vi "Get Key-Value Pairs from Attribute List.vi"(7 "element name (for errors)":string, 8 "error in (no error)":errorcluster, 10 "attribute list":string) -> (0 "error out":errorcluster, 2 "attributes":cluster{"name":string[], "value":string[]})   [LabVIEW 2011]
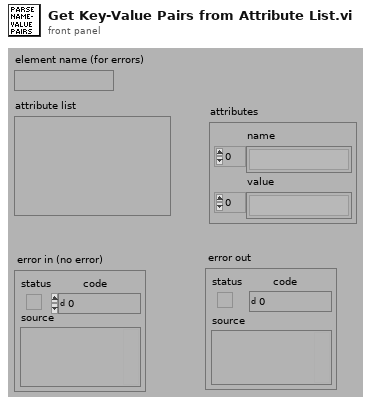
[diagram p1: front panel]
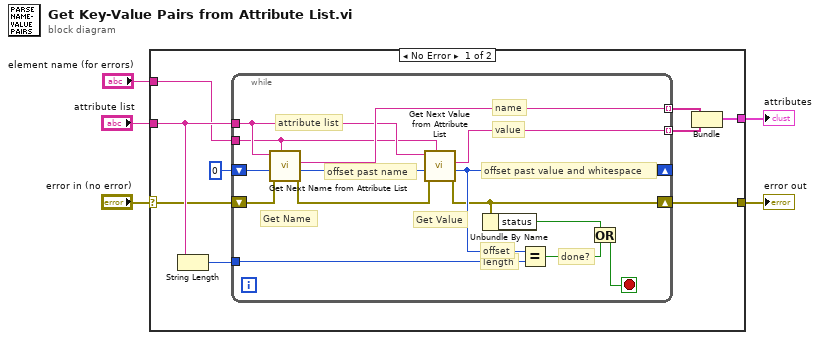
[diagram p0: block diagram]
diagram:
  n1 = case shown="No Error" "error in (no error)" {
    selector: "error in (no error)" -> [w7 w29]
    tunnel: [w14 _] -> w5
    tunnel: "attribute list" -> [w12 _]
    tunnel: [w11 w29] -> w3
    tunnel: "element name (for errors)" -> [w6 _]
    frame No Error {
      n2 = String Length(string=w12) -> (length=w8:i32)
      n3 = while {
        tunnel: [w24] -> w10 mode=indexing
        tunnel: w12 -> [w18]
        tunnel: [w19] -> w13 mode=indexing
        shift-right: [w28] -> _
        shift-left: 0 ("offset past match") -> [w23]
        tunnel: w8 -> [w27]
        shift-right: [w17] -> w11
        shift-left: w7 -> [w21]
        tunnel: w6 -> [w15]
        stop <- w25 stop-if-true
        # "attribute list"
        # "offset"
        # "length"
        # "done?"
        # "offset past value and whitespace"
        # "offset past name"
        # "value"
        # "Get Value"
        # "name"
        # "Get Name"
        n4 = call "Get Next Name from Attribute List.vi"("element name (for errors)"=w15, "error in"=w21, "offset"=w23, "attribute list"=w18) -> ("error out"=w20:errorcluster, "offset past name"=w22:i32, "name"=w24:string)  [unwired: 5 in]
        n5 = call "Get Next Value from Attribute List.vi"("element name (for errors)"=w15, "error in"=w20, "offset"=w22, "attribute list"=w18) -> ("error out"=w17:errorcluster, "offset past value and whitespace"=w28:i32, "value"=w19:string)  [unwired: 5 in]
        n6 = Unbundle By Name(w17) -> ("status"=w16:bool)
        n7 = Equal?(x=w28, y=w27) -> (x = y?=w26:bool)
        n8 = Or(x=w16, y=w26) -> (x .or. y?=w25:bool)
      }
      n9 = Bundle(w10, w13) -> (w14:cluster{string[], string[]})  [unwired: 1 in]
    }
    frame Error {
    }
  }
  "attributes" <- w5
  "error out" <- w3
